vi "WriteHeader.vi"(8 "Error in":errorcluster) -> (0 "Error out":errorcluster, 2 "Header string array":string[](array[string]))   [LabVIEW 2017, in "LeapMotion.lvlib"]
uses:
  LeapMotion.lvlib
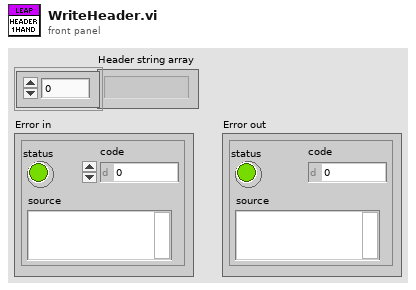
[diagram p1: front panel]
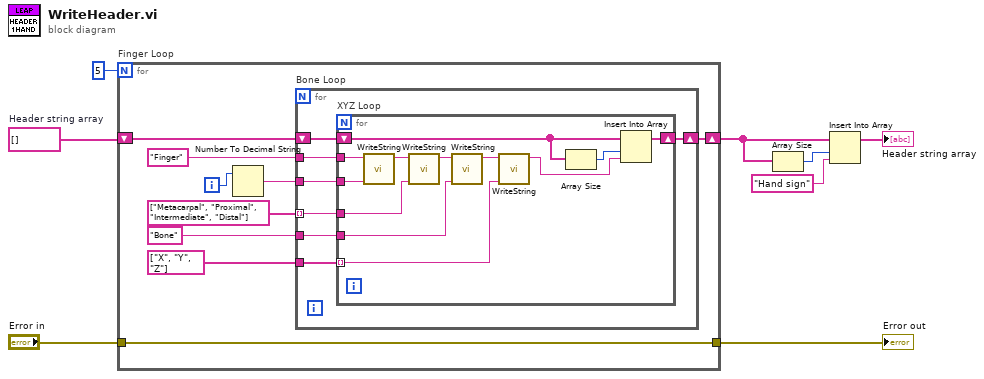
[diagram p0: block diagram]
diagram:
  w4 = string[] []  # Header string array
  n1 = for "Finger Loop" {
    N: 5 -> [_]
    shift-right: [w17] -> w7
    shift-left: w4 -> [w13]
    tunnel: "Error in" -> [w9]
    tunnel: [w9] -> w2
    i -> [w16]
    n2 = Number To Decimal String(number=w16) -> (decimal integer string=w10:string)  [unwired: 1 in]
    n3 = for "Bone Loop" {
      tunnel: string[] ["Metacarpal", "Proximal", "Intermediate", "Distal"] ("Bone name") -> [w21] mode=indexing
      tunnel: string[] ["X", "Y", "Z"] ("Dimension") -> [w22]
      shift-right: [w23] -> w17
      shift-left: w13 -> [w24]
      tunnel: "Bone" -> [w20]
      tunnel: "Finger" -> [w19]
      tunnel: w10 -> [w18]
      n4 = for "XYZ Loop" {
        tunnel: w22 -> [w28] mode=indexing
        shift-right: [w36] -> w23
        shift-left: w24 -> [w35]
        tunnel: w21 -> [w31]
        tunnel: w20 -> [w29]
        tunnel: w19 -> [w33]
        tunnel: w18 -> [w26]
        n5 = call "WriteString.vi"("To apppend"=w26, "Original string"=w33) -> ("Appended string"=w32:string)  [unwired: 9 in]
        n6 = call "WriteString.vi"("To apppend"=w31, "Original string"=w32) -> ("Appended string"=w30:string)  [unwired: 9 in]
        n7 = call "WriteString.vi"("To apppend"=w29, "Original string"=w30) -> ("Appended string"=w27:string)  [unwired: 9 in]
        n8 = call "WriteString.vi"("To apppend"=w28, "Original string"=w27) -> ("Appended string"=w25:string)  [unwired: 9 in]
        n9 = Array Size(array=w35) -> (size(s)=w34:i32)
        n10 = Insert Into Array(array=w35, index=w34, new element=w25) -> (w36:string[])
      }
    }
  }
  "Error out" <- w2
  n11 = Array Size(array=w7) -> (size(s)=w6:i32)
  n12 = Insert Into Array(array=w7, index=w6, new element="Hand sign") -> (→"Header string array":string[])
